vi "文件路径.vi"(10 "文件路径":path, 11 "文件格式":string=".BMP") -> (2 "新路径":path)   [LabVIEW 2018]
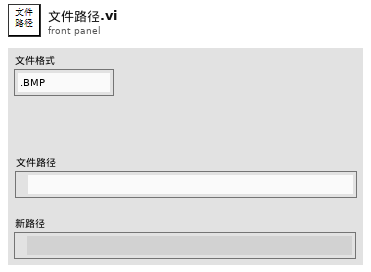
[diagram p1: front panel]
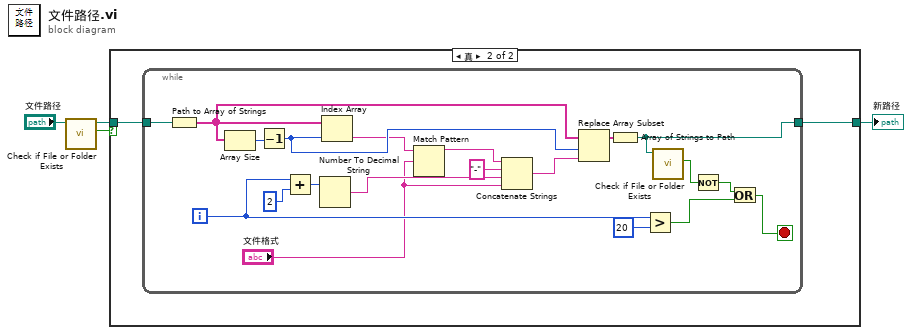
[diagram p0: block diagram]
diagram:
  n1 = call <vilib>:"Check if File or Folder Exists.vi"("path"="文件路径") -> ("file or folder exists?"=w3:bool, "dup path"=w2:path)  [unwired: 8 in, 1 out]
  n2 = case shown="真" w3 {
    tunnel: w2 -> [w5 w7]
    tunnel: [w5 w6] -> w1
    frame False {
    }
    frame True {
      n3 = while {
        tunnel: w7 -> [w22]
        tunnel: [w20] -> w6
        i -> [w18]
        stop <- w19 stop-if-true
        n4 = Path to Array of Strings(0:w22) -> (2:w21:string[])  [unwired: 1 out]
        n5 = Array Size(array=w21) -> (size(s)=w27:i32)
        n6 = Decrement(x=w27) -> (x-1=w26:i32)
        n7 = Add(x=w18, y=2) -> (x+y=w24:i32)
        n8 = Number To Decimal String(number=w24) -> (decimal integer string=w10:string)  [unwired: 1 in]
        n9 = Index Array(array=w21, index=w26) -> (element=w13:string)
        n10 = Match Pattern(string=w13, regular expression="文件格式") -> (before substring=w12:string)  [unwired: 1 in, 3 out]
        n11 = Concatenate Strings(w12, "-" ("字符串"), w10, "文件格式") -> (w9:string)
        n12 = Replace Array Subset(array=w21, new element=w9, index=w26) -> (w23:string[])
        n13 = Array of Strings to Path(0:w23) -> (2:w20:path)  [unwired: 1 in]
        n14 = Greater?(x=w18, y=20) -> (0:w17:bool)
        n15 = call <vilib>:"Check if File or Folder Exists.vi"("path"=w20) -> ("file or folder exists?"=w14:bool)  [unwired: 8 in, 2 out]
        n16 = Not(x=w14) -> (.not. x?=w15:bool)
        n17 = Or(x=w15, y=w17) -> (x .or. y?=w19:bool)
      }
    }
  }
  "新路径" <- w1
